vi "Wait For Response.vi"(8 "error in (no error)":errorcluster, 11 "HttpResponseMessage in":refnum<class "HttpResponseMessage.lvclass">) -> (0 "error out":errorcluster, 1 "TaskIsCompleted":bool, 2 "TaskStatus":i32(ring) items=["Created", "WaitingForActivation", "WaitingToRun", "Running", "WaitingForChildrenToComplete", "RanToCompletion", "Canceled", "Faulted"], 3 "HttpResponseMessage out":refnum<class "HttpResponseMessage.lvclass">, 4 "TaskTimeout":bool)   [LabVIEW 2018, in "HttpClient_NET.lvlib" / "HttpResponseMessage.lvclass"]
doc: "<b> </b> <b> </b>\nHttpClient_NET\nJustin Young - Viviota\nCopyright (c) 2021\nLicense: BSD"
uses:
  HttpResponseMessage.lvclass
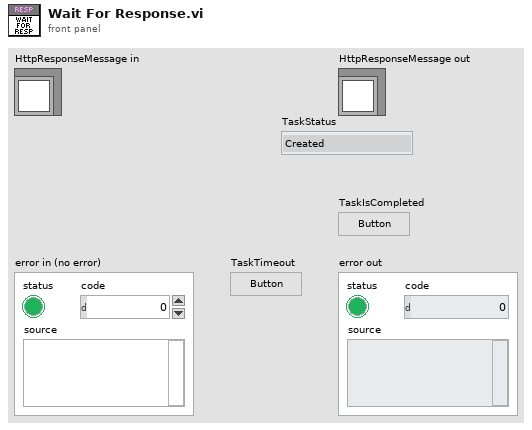
[diagram p1: front panel]
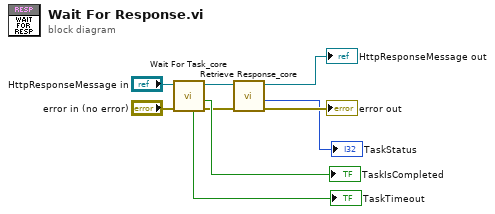
[diagram p0: block diagram]
diagram:
  n1 = call "Wait For Task_core.vi"("error in (no error)"="error in (no error)", "HttpResponseMessage in"="HttpResponseMessage in") -> ("error out"=w6:errorcluster, "IsCompleted"=→"TaskIsCompleted":bool, "HttpResponseMessage out"=w3:refnum<class "HttpResponseMessage.lvclass">, "Timeout"=→"TaskTimeout":bool)  [unwired: 6 in]
  n2 = call "Retrieve Response_core.vi"("error in (no error)"=w6, "HttpResponseMessage in"=w3) -> ("error out"=→"error out":errorcluster, "Status"=→"TaskStatus":i32, "HttpResponseMessage out"=→"HttpResponseMessage out":refnum<class "HttpResponseMessage.lvclass">)  [unwired: 6 in, 1 out]
